vi "Save Configuration.vi"(8 "error in (no error)":errorcluster, 11 "VISA resource name":refnum<visa-resource-name>) -> (0 "error out":errorcluster, 3 "VISA resource name out":refnum<visa-resource-name>)   [LabVIEW 2018, in "XP Power PLS600.lvlib"]
doc: "Saves configuration parameters to non-volatile memory. Contents consist of:\n\n• Analog Current Scaling Select (3V/5V/10V)\n• Analog Voltage Scaling Select (3V/5V/10V)\n• Auto-Start (Enabled/Disabled)\n• Calibrated Flag (Calibrated/Not Calibrated)\n• Control Source (Local/Remote/Remote with Lock/Analog Voltage Control/Analog Current Control/Analog Dual Control)\n• Conversion Current Raw-to-User Slope and Intercept\n• Conversion Voltage Raw-to-User Slope and Intercept\n• Model\n• Over-Current Protection Level\n• Over-Power Protection Level\n• Over-Voltage Protection Level\n• Remote Sense (Enabled/Disabled)\n• Remote Sense Lead Resistance\n• Unit Serial Number\n\nThis command can be executed from any of the six operating modes (Local, Remote, Remote with Lock, Analog Voltage Control, Analog Current Control, or Analog Dual Control) or during Remote Calibration, but only when the output is deactivated."
uses:
  XP Power PLS600.lvlib
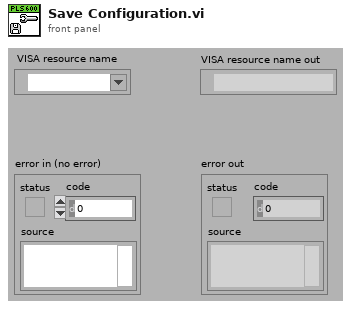
[diagram p1: front panel]
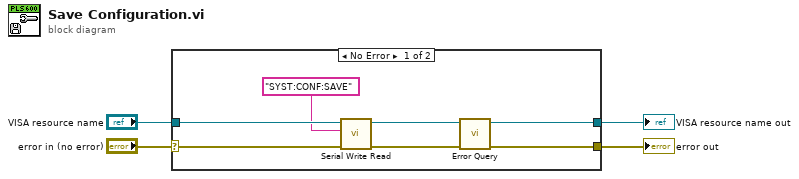
[diagram p0: block diagram]
diagram:
  n1 = case shown="No Error" "error in (no error)" {
    selector: "error in (no error)" -> [w6 w13]
    tunnel: [w11 w12] -> w4
    tunnel: [w10 w13] -> w3
    tunnel: "VISA resource name" -> [w9 w12]
    frame No Error {
      n2 = call "Serial Write Read.vi"("error in (no error)"=w6, "Write Buffer"="SYST:CONF:SAVE", "VISA resource name"=w9) -> ("error out"=w5:errorcluster, "VISA resource name out"=w7:refnum<visa-resource-name>)  [unwired: 6 in, 1 out]
      n3 = call "Error Query.vi"("error in (no error)"=w5, "VISA resource name"=w7) -> ("error out"=w10:errorcluster, "VISA resource name out"=w11:refnum<visa-resource-name>)  [unwired: 6 in, 2 out]
    }
    frame Error {
    }
  }
  "VISA resource name out" <- w4
  "error out" <- w3
